vi "niDTS WLAN INSTR TX WaitOnIdle.vi"(8 "error in (no error)":errorcluster, 9 "Result Instance":i32=1, 10 "Driver Instance":i32=1, 11 "niDTS WLAN INSTR TX in":refnum<class "niDTS WLAN INSTR TX.lvclass">) -> (0 "error out":errorcluster, 3 "niDTS WLAN INSTR TX out":refnum<class "niDTS WLAN INSTR TX.lvclass">)   [LabVIEW 2015, in "niDTS WLAN.lvlib" / "niDTS WLAN INSTR TX.lvclass"]
uses:
  niDTS WLAN INSTR TX.lvclass
  niDTS WLAN INSTR TX.lvclass/niDTS WLAN INSTR TX.ctl
  RiviInstDriver/InstDriver/Objects/InstDriver.lvclass
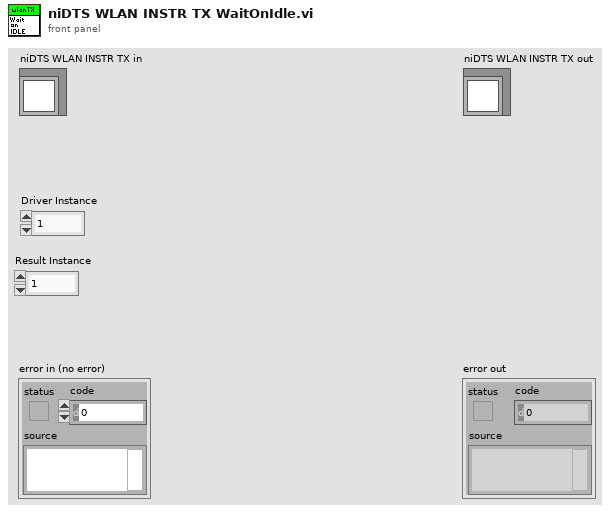
[diagram p1: front panel]
types:
  T1 = typedef "niRfsaWlan.lvclass/niRfsaWlan INC Handle.ctl" = refnum<data-value>
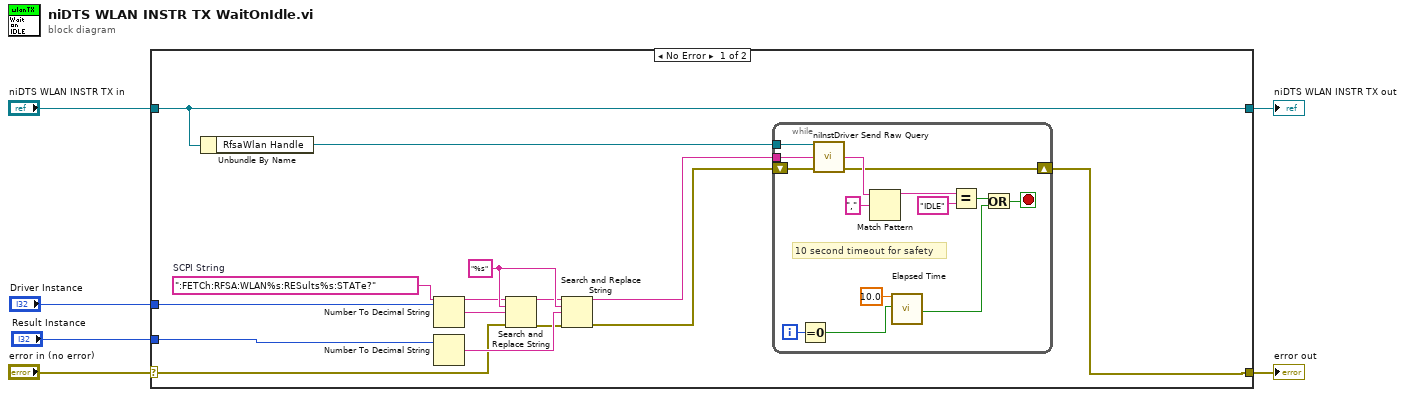
[diagram p0: block diagram]
diagram:
  n1 = case shown="No Error" "error in (no error)" {
    selector: "error in (no error)" -> [w11 w36]
    tunnel: [w7 w36] -> w5
    tunnel: [w20 w35] -> w3
    tunnel: "niDTS WLAN INSTR TX in" -> [w20 w35]
    tunnel: "Driver Instance" -> [w13 _]
    tunnel: "Result Instance" -> [w12 _]
    frame No Error {
      w16 = "%s" ("search string")
      w14 = ":FETCh:RFSA:WLAN%s:RESults%s:STATe?"  # SCPI String
      n2 = Unbundle By Name(w20) -> ("RfsaWlan Handle"=w10:T1)
      n3 = Number To Decimal String(number=w13) -> (decimal integer string=w18:string)  [unwired: 1 in]
      n4 = Number To Decimal String(number=w12) -> (decimal integer string=w19:string)  [unwired: 1 in]
      n5 = Search and Replace String(input string=w14, search string=w16, replace string=w18, error in=w11) -> (result string=w15:string, error out=w17:errorcluster)  [unwired: 4 in, 2 out]
      n6 = Search and Replace String(input string=w15, search string=w16, replace string=w19, error in=w17) -> (result string=w9:string, error out=w8:errorcluster)  [unwired: 4 in, 2 out]
      n7 = while {
        tunnel: w10 -> [w34]
        tunnel: w9 -> [w33]
        shift-right: [w21] -> w7
        shift-left: w8 -> [w32]
        i -> [w25]
        stop <- w26 stop-if-true
        # "10 second timeout for safety"
        n8 = Equal To 0?(x=w25) -> (x = 0?=w24:bool)
        n9 = call "niInstDriver Send Raw Query.vi"("InstDriver Handle in"=w34, "Query"=w33, "error in (no error)"=w32) -> ("Response"=w28:string, "error out"=w21:errorcluster)  [unwired: 10 in, 1 out]
        n10 = Match Pattern(string=w28, regular expression=",") -> (before substring=w30:string)  [unwired: 1 in, 3 out]
        n11 = call "Elapsed Time"("Time Target (s)"=10.0, "Reset"=w24) -> ("Time has Elapsed"=w22:bool)  [unwired: 10 in, 7 out]
        n12 = Equal?(x=w30, y="IDLE") -> (x = y?=w27:bool)
        n13 = Or(x=w27, y=w22) -> (x .or. y?=w26:bool)
      }
    }
    frame Error {
    }
  }
  "error out" <- w5
  "niDTS WLAN INSTR TX out" <- w3
